vi "instantiate_text_file_source.vi"(0 "source_folder":path, 5 "file_extension":string, 7 "recursive_folder_load":bool, 11 "error in (no error)":errorcluster) -> (4 "datasource_text_file out":refnum<class "datasource_text_file.lvclass">, 15 "error out":errorcluster)   [LabVIEW 2020, in "datasource_text_file.lvclass"]
uses:
  datasource_text_file.lvclass
  datasource_text_file.lvclass/datasource_text_file.ctl
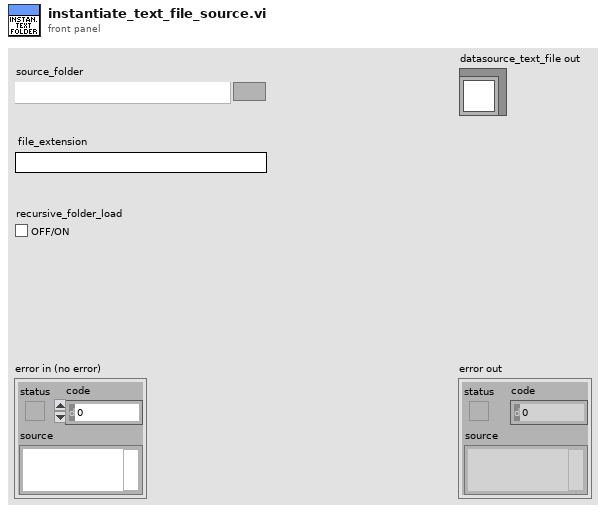
[diagram p1: front panel]
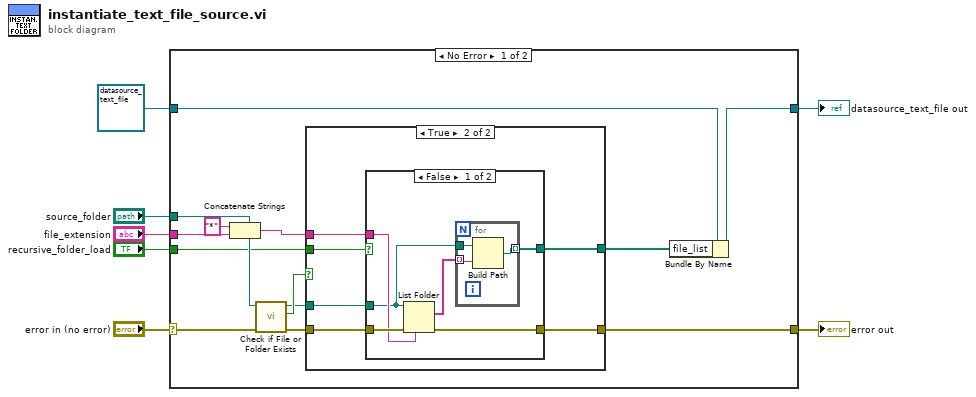
[diagram p0: block diagram]
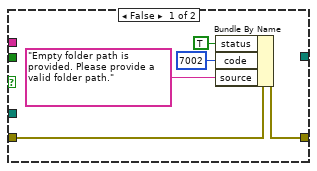
[diagram p2: hidden frame]
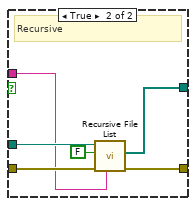
[diagram p3: hidden frame]
diagram:
  n1 = case shown="No Error" "error in (no error)" {
    selector: "error in (no error)" -> [w20 w48]
    tunnel: [w15 w48] -> w6
    tunnel: [w10 w47] -> w4
    tunnel: refnum<class "datasource_text_file.lvclass"> refnum ("datasource_text_file in") -> [w12 w47]
    tunnel: "source_folder" -> [w19 _]
    tunnel: "file_extension" -> [w14 _]
    tunnel: "recursive_folder_load" -> [w13 _]
    frame No Error {
      n2 = Concatenate Strings("*" ("string"), w14) -> (w9:string)
      n3 = call <vilib>:"Check if File or Folder Exists.vi"("error in (no error)"=w20, "path"=w19) -> ("error out"=w16:errorcluster, "file or folder exists?"=w18:bool, "dup path"=w17:path)  [unwired: 7 in]
      n4 = case shown="True" w18 {
        tunnel: w17 -> [_ w31]
        tunnel: w16 -> [w25 w30]
        tunnel: [w24 w29] -> w15
        tunnel: w9 -> [_ w28]
        tunnel: w13 -> [_ w27]
        tunnel: [_ w26] -> w11
        frame False {
          n5 = Bundle By Name(cluster=w25, "status"=TRUE, "code"=7002, "source"="Empty folder path is provided. Please provide a valid folder path.") -> (w24:errorcluster)
        }
        frame True {
          n6 = case shown="False" w27 {
            tunnel: w31 -> [w33 w46]
            tunnel: w30 -> [w37 w45]
            tunnel: [w36 w44] -> w29
            tunnel: w28 -> [w35 w42]
            tunnel: [w32 w41] -> w26
            frame False {
              n7 = List Folder(path=w33, pattern=w35, error in=w37) -> (filenames=w34:string[], error out=w36:errorcluster)  [unwired: 1 in, 2 out]
              n8 = for {
                tunnel: w34 -> [w39] mode=indexing
                tunnel: w33 -> [w40]
                tunnel: [w38] -> w32 mode=indexing
                n9 = Build Path(base path=w40, name or relative path=w39) -> (appended path=w38:path)
              }
            }
            frame True {
              # "Recursive"
              n10 = call <vilib>:"Recursive File List.vi"("pattern"=w42, "error in (no error)"=w45, "Treat LLBs as Folders?"=FALSE, "Folder Path"=w46) -> ("error out"=w44:errorcluster, "All Files in Dir"=w41:path[])  [unwired: 3 in, 3 out]
            }
          }
        }
      }
      n11 = Bundle By Name(cluster=w12, "file_list"=w11) -> (w10:refnum<class "datasource_text_file.lvclass">)
    }
    frame Error {
    }
  }
  "error out" <- w6
  "datasource_text_file out" <- w4
